vi "Edit Text File.vi"(8 "error in (no error)":errorcluster, 11 "file path":path) -> (0 "error out":errorcluster)   [LabVIEW 2019, in "Build.lvlib"]
uses:
  Build.lvlib
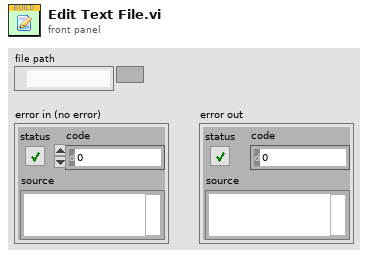
[diagram p1: front panel]
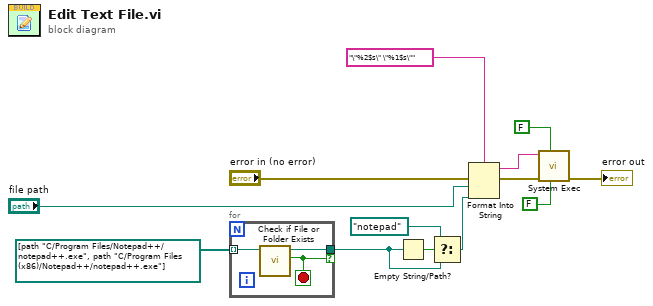
[diagram p0: block diagram]
diagram:
  n1 = for {
    tunnel: [w16] -> w11 if=w15
    tunnel: path[] [path "C:/Program Files/Notepad++/notepad++.exe", path "C:/Program Files (x86)/Notepad++/notepad++.exe"] ("path") -> [w14] mode=indexing
    stop <- w15 stop-if-true
    n2 = call <vilib>:"Check if File or Folder Exists.vi"("path"=w14) -> ("file or folder exists?"=w15:bool, "dup path"=w16:path)  [unwired: 8 in, 1 out]
  }
  n3 = Empty String/Path?(string/path=w11) -> (empty?=w10:bool)
  n4 = Select(t=path "notepad", s=w10, f=w11) -> (s? t:f=w12:path)
  n5 = Format Into String(format string="\"%2$s\" \"%1$s\"", error in="error in (no error)", "file path", w12) -> (resulting string=w4:string, error out=w6:errorcluster)  [unwired: 1 in]
  n6 = call <vilib>:"System Exec.vi"("run minimized? (F)"=FALSE, "wait until completion? (T)"=FALSE, "error in (no error)"=w6, "command line"=w4) -> ("error out"=→"error out":errorcluster)  [unwired: 4 in, 3 out]
